vi "set_logic_statement.vi"(8 "error in (no error)":errorcluster, 9 "statement":string, 10 "statement number":u8, 11 "VISA resource name":refnum<visa-resource-name>) -> (0 "error out":errorcluster, 3 "VISA resource name out":refnum<visa-resource-name>)   [LabVIEW 2018]
doc: "Update a logic statement."
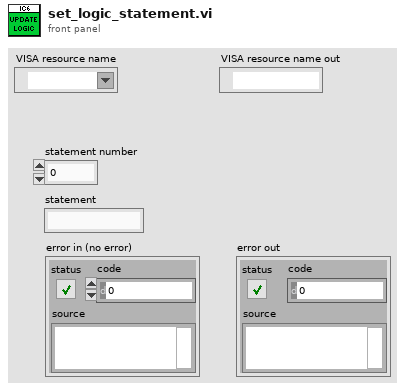
[diagram p1: front panel]
types:
  T1 = enum16{"Source", "General", "Input name", "Process name", "Logic", "Material", "Material name", "Output name", "Process", "Sensor", "Output type", "User message", "Layer", ""}
  T2 = enum16{"Hello", "Query", "Remote action", "Status", "Update"}
  T3 = cluster{"statement number":u8, "statement":string}
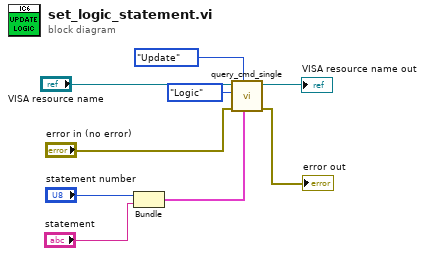
[diagram p0: block diagram]
diagram:
  n1 = Bundle("statement number"="statement number", "statement"="statement") -> (w3:T3)  [unwired: 1 in]
  n2 = call "query_cmd_single.vi"("Parameter"=w3, "Command group"=T2."Update", "error in (no error)"="error in (no error)", "Command subgroup"=T1."Logic", "VISA resource name"="VISA resource name") -> ("error out"=→"error out":errorcluster, "VISA resource name out"=→"VISA resource name out":refnum<visa-resource-name>)  [unwired: 2 in, 3 out]
